vi "Get_processed beam data.vi"(0 "Beam in":refnum<class "Beam.lvclass">, 5 "error in (no error)":errorcluster) -> (14 "Beam out":refnum<class "Beam.lvclass">, 15 "Spill ID":dbl, 16 "Recent spill Intensity":dbl, 17 "Acumilated Intensity":dbl, 18 "Spil Counter":dbl, 19 "error out":errorcluster)   [LabVIEW 2019, in "Beam.lvclass"]
uses:
  Beam.lvclass
  Beam.lvclass/Beam.ctl
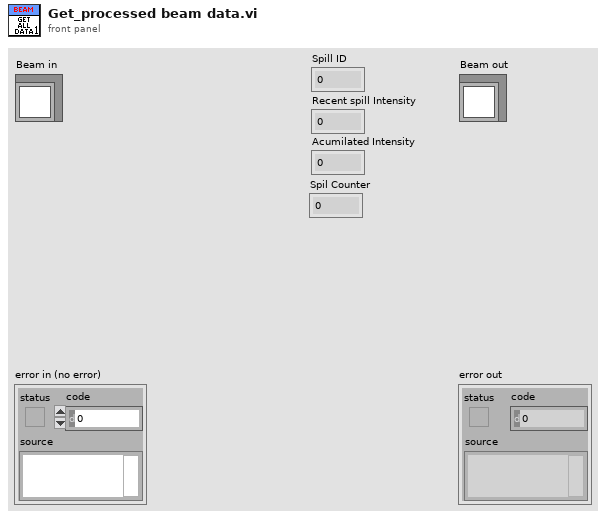
[diagram p1: front panel]
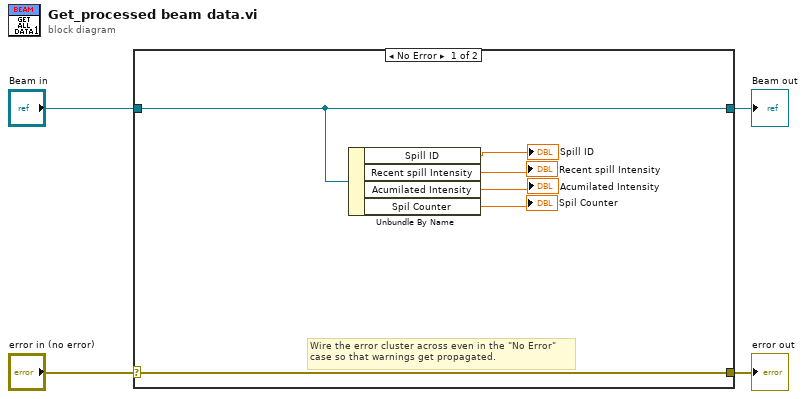
[diagram p0: block diagram]
diagram:
  n1 = case shown="No Error" "error in (no error)" {
    selector: "error in (no error)" -> [w10 w12]
    tunnel: [w10 w12] -> w3
    tunnel: [w9 w11] -> w1
    tunnel: "Beam in" -> [w9 w11]
    frame No Error {
      # "Wire the error cluster across even in the \"No Error\"\ncase so that warnings get propagated."
      n2 = Unbundle By Name(w9) -> ("Spill ID"=→"Spill ID":dbl, "Recent spill Intensity"=→"Recent spill Intensity":dbl, "Acumilated Intensity"=→"Acumilated Intensity":dbl, "Spil Counter"=→"Spil Counter":dbl)
    }
    frame Error {
    }
  }
  "error out" <- w3
  "Beam out" <- w1
